vi "M300.vi"() -> ()   [LabVIEW 2014]
uses:
  <vilib>/Waveform/DWDTOps.llb/DWDT Binary U32 to Digital.vi
  <vilib>/Waveform/DWDTOps.llb/DWDT Digital to Analog.vi
panel:
  in  "line index":i32
  out "analog waveform":waveform(dbl)
  out "digital waveform":digitalwaveform(waveform)
  in  "error out":errorcluster
  in  "?":bool
  out "Overall Minimum Voltage":dbl format="%#_8g"
  out "Overall Maximum Voltage":dbl format="%#_8g"
  out "Voltage String":string
  out "Voltage":dbl format="%#_8g"
  in  "VISA resource name":refnum<visa-resource-name>
  in  "Boolean":bool=TRUE
  in  "error in (no error)":errorcluster
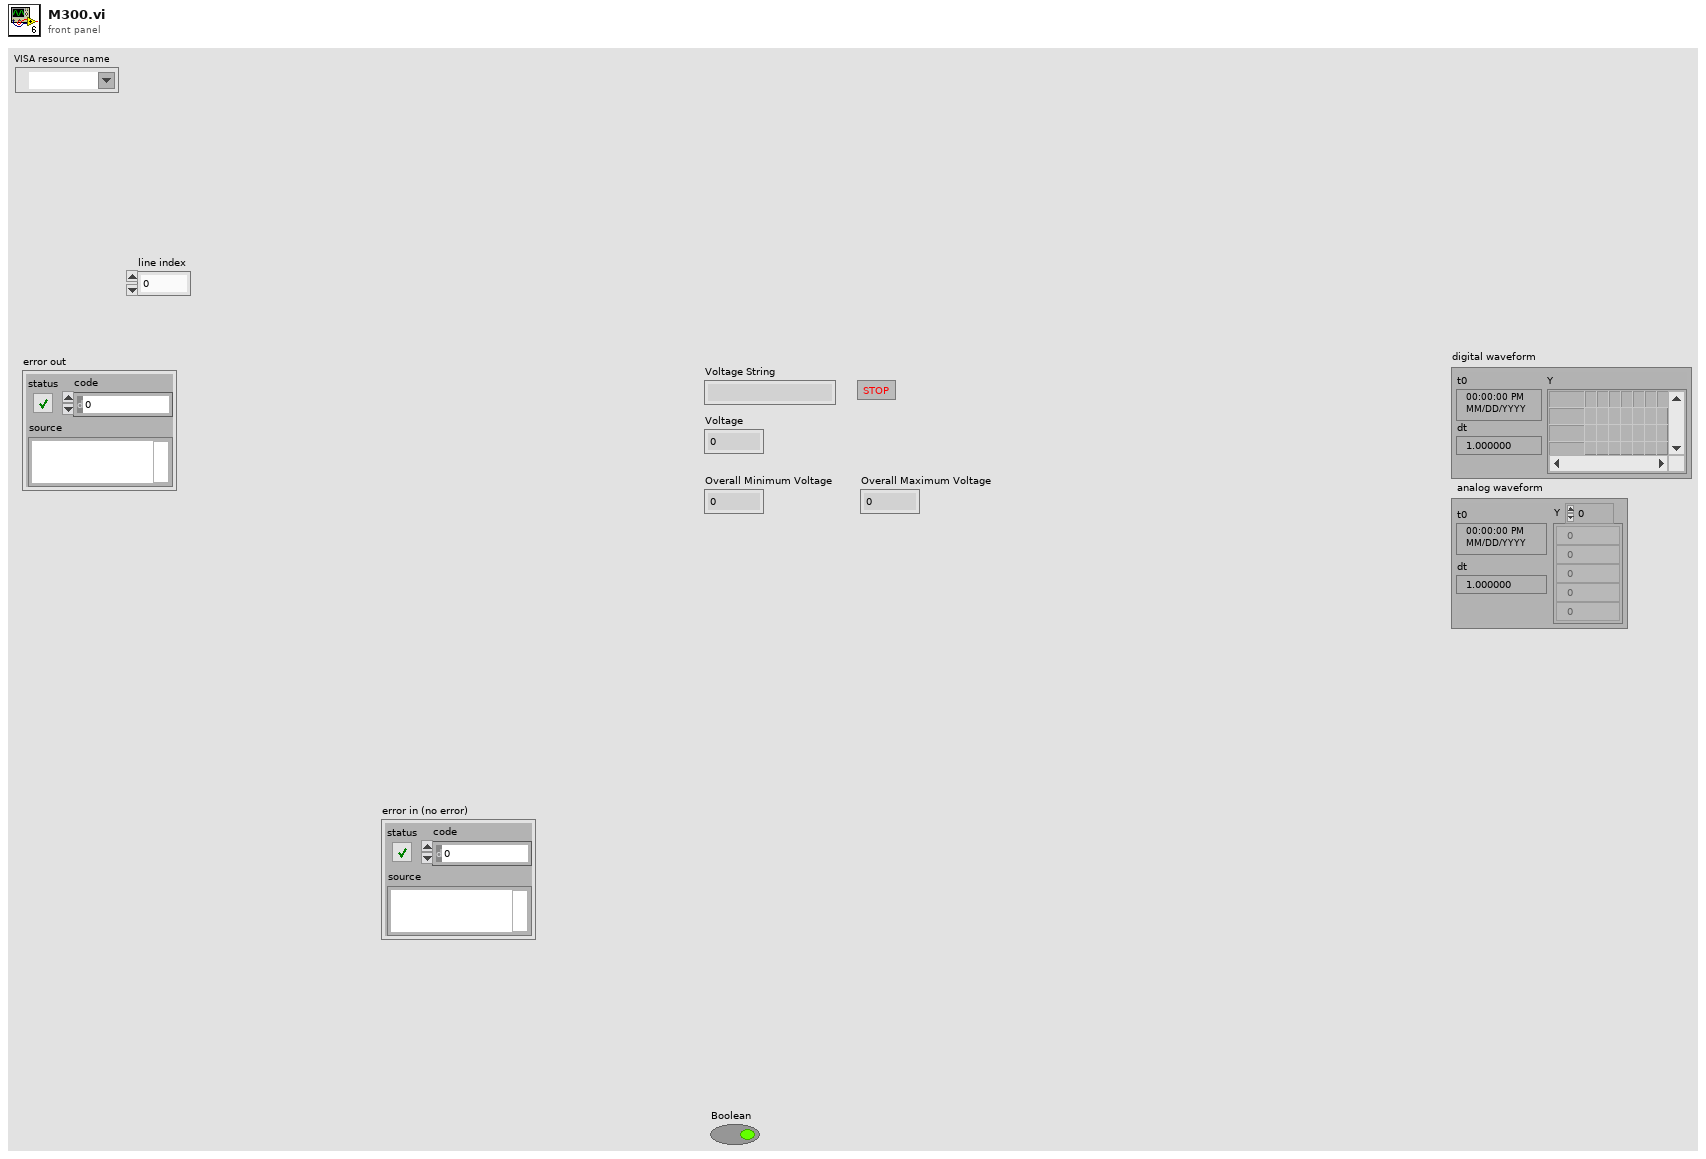
[diagram p1: front panel]
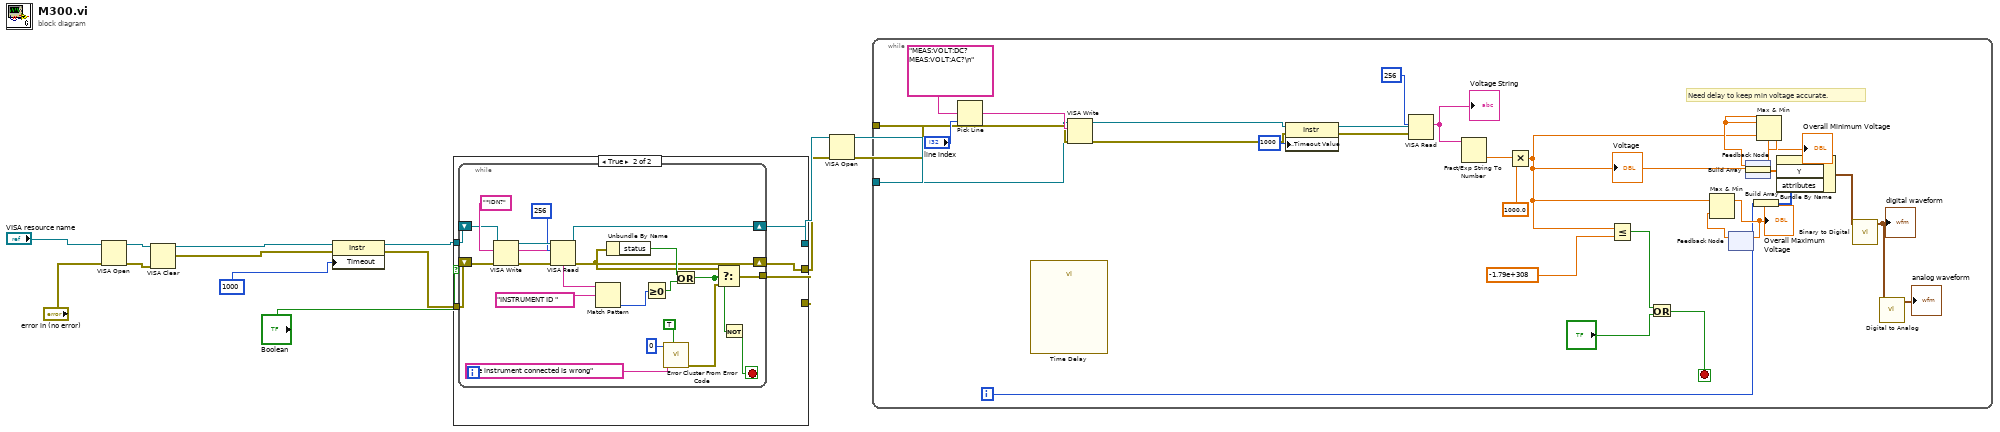
[diagram p0: block diagram]
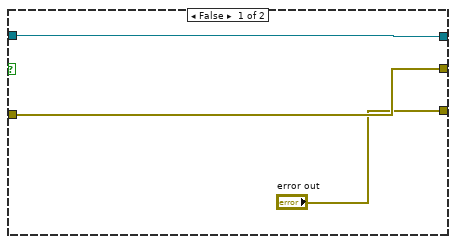
[diagram p2: hidden frame]
diagram:
  n1 = VISA Open(error in (no error)="error in (no error)", VISA resource name="VISA resource name") -> (VISA resource name=w12:refnum<visa-resource-name>, error out=w11:errorcluster)  [unwired: 3 in]
  n2 = VISA Clear(VISA resource name=w12, error in (no error)=w11) -> (VISA resource name out=w10:refnum<visa-resource-name>, error out=w9:errorcluster)
  n3 = property class="Instr"(reference=w10, error in=w9, "Timeout"=u32 1000 ("General Settings:Timeout Value")) -> (reference out=w7:refnum<visa-resource-name>, error out=w6:errorcluster)
  n4 = case shown="True" "Boolean" {
    tunnel: w7 -> [w17 w22]
    tunnel: w6 -> [w16 w21]
    tunnel: [w17 w20] -> w4
    tunnel: [w16 w19] -> w2
    tunnel: ["error out" w18] -> _
    frame False {
    }
    frame True {
      n5 = while {
        shift-right: [w29] -> w20
        shift-left: w22 -> [w31]
        shift-right: [w28] -> w19
        shift-left: w21 -> [w30]
        tunnel: [w26] -> w18
        stop <- w23 stop-if-true
        w32 = "*IDN?" ("instrument ID")
        n6 = VISA Write(VISA resource name=w31, write buffer=w32, error in (no error)=w30) -> (VISA resource name out=w41:refnum<visa-resource-name>, error out=w40:errorcluster)  [unwired: 1 out]
        n7 = VISA Read(VISA resource name=w41, byte count=u32 256, error in (no error)=w40) -> (VISA resource name out=w29:refnum<visa-resource-name>, error out=w28:errorcluster)  [unwired: 2 out]
        n8 = Match Pattern(string=w32, regular expression="INSTRUMENT ID ") -> (offset past match=w37:i32)  [unwired: 1 in, 3 out]
        n9 = Unbundle By Name(w28) -> ("status"=w35:bool)
        n10 = Greater Or Equal To 0?(x=w37) -> (x >= 0?=w36:bool)
        n11 = call <vilib>:"Error Cluster From Error Code.vi"("show call chain? (False)"=TRUE, "error message (\"\")"="The instrument connected is wrong" ("error message (\"\")"), "error code (0)"=0) -> ("error out"=w25:errorcluster)  [unwired: 6 in]
        n12 = Or(x=w35, y=w36) -> (x .or. y?=w24:bool)
        n13 = Select(t=w28, s=w24, f=w25) -> (s? t:f=w26:errorcluster)
        n14 = Not(x=w24) -> (.not. x?=w23:bool)
      }
    }
  }
  n15 = VISA Open(error in (no error)=w2, VISA resource name=w4) -> (VISA resource name=w3:refnum<visa-resource-name>, error out=w1:errorcluster)  [unwired: 3 in]
  n16 = while {
    tunnel: w3 -> [w48]
    tunnel: w1 -> [w49]
    i -> [w57]
    stop <- w60 stop-if-true
    # "Need delay to keep min voltage accurate."
    n17 = Pick Line(multi-line string="MEAS:VOLT:DC? MEAS:VOLT:AC?\n" ("function"), line index="line index") -> (output string=w50:string)  [unwired: 1 in]
    n18 = call "Time Delay"() -> ()  [unwired: 11 in, 1 out]
    n19 = VISA Write(VISA resource name=w48, write buffer=w50, error in (no error)=w49) -> (VISA resource name out=w43:refnum<visa-resource-name>, error out=w42:errorcluster)  [unwired: 1 out]
    n20 = property class="Instr"(reference=w43, error in=w42, "General Settings:Timeout Value"=u32 1000) -> (reference out=w45:refnum<visa-resource-name>, error out=w44:errorcluster)
    n21 = VISA Read(VISA resource name=w45, byte count=u32 256, error in (no error)=w44) -> (read buffer=w68:string)  [unwired: 3 out]
    "Voltage String" <- w68
    n22 = Fract/Exp String To Number(string=w68) -> (number=w70:dbl)  [unwired: 3 in, 1 out]
    n23 = Multiply(x=w70, y=1000.0) -> (x*y=w58:dbl)
    "Voltage" <- w58
    n24 = Less Or Equal?(x=w58, y=-1.79e+308) -> (x <= y?=w66:bool)
    n25 = Or(x=w66, y="?") -> (x .or. y?=w60:bool)
    n26 = feedback #1() -> (w63:dbl)  [unwired: 1 in]
    n27 = Max & Min(x=w58, y=w63) -> (max(x,y)=w62:dbl)  [unwired: 1 out]
    "Overall Maximum Voltage" <- w62
    n28 = feedback-in #1(w62) -> ()
    n29 = feedback #2() -> (w61:dbl)  [unwired: 1 in]
    "Overall Minimum Voltage" <- w61
    n30 = Build Array(w58) -> (w59:dbl[])
    n31 = Build Array(w57) -> (w56:i32[])
    n32 = Max & Min(x=w61, y=w58) -> (min(x,y)=w64:dbl)  [unwired: 1 out]
    n33 = feedback-in #2(w64) -> ()
    n34 = Bundle By Name("Y"=w59, "attributes"=w56) -> (w55:waveform(dbl))  [unwired: 1 in]
    n35 = call-poly <vilib>:"Binary to Digital.vi"("binary array"=w55) -> ("digital waveform"=w54:digitalwaveform)  [unwired: 9 in, 1 out]
    "digital waveform" <- w54
    n36 = call-poly <vilib>:"Digital to Analog.vi"("digital waveform"=w54) -> ("analog waveform"=→"analog waveform":waveform(dbl))  [unwired: 7 in, 3 out]
  }
